vi "To String.vi"(11 "JSON String in":refnum<class "JSON String.lvclass">) -> (2 "String":string)   [LabVIEW 2017, in "LVJSON.lvlib" / "JSON String.lvclass"]
uses:
  JSON String.lvclass
  JSON String.lvclass/JSON String.ctl
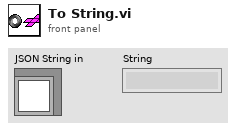
[diagram p1: front panel]
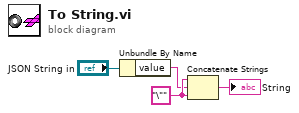
[diagram p0: block diagram]
diagram:
  w3 = "\"" ("string")
  n1 = Unbundle By Name("JSON String in") -> ("value"=w2:string)
  n2 = Concatenate Strings(w3, w2, w3) -> (→"String":string)
